vi "Camera Loop.vi"(6 "Used functions":bool=TRUE, 8 "error in":errorcluster, 9 "IBM OptoElectroMechanics Configuration":T1={"Parameter Analizer"={"Parameter Analyzer VISA Session"="COM1", "Sweeping Time Parameters"={"Integration Time"=0, "Short Integration Time (s)"=1.0, "Long Integration Time (s)"=0.0, "Wait Time Parameter"=1.0}, "Acquisition Mode"=enum."Sweeping Mode", "Status Polling Time (ms)"=0, "Comment"="Test VI", "SMU 1 - Sweeping"={"Start / Offset"=0.0, "Stop / Ratio"=1.0, "Step \n(linear only)"=0.01, "Compliance"=0.1, "Power \nCompliance"=0.0, "Mode"=0, "Function"=0, "Sweep Mode"=FALSE}, "SMU 2 - Sweeping"={"Start / Offset"=0.0, "Stop / Ratio"=1.0, "Step \n(linear only)"=0.01, "Compliance"=0.1, "Power \nCompliance"=0.0, "Mode"=0, "Function"=0, "Sweep Mode"=FALSE}, "SMU 3 - Sweeping"={"Start / Offset"=0.0, "Stop / Ratio"=1.0, "Step \n(linear only)"=0.01, "Compliance"=0.1, "Power \nCompliance"=0.0, "Mode"=0, "Function"=0, "Sweep Mode"=FALSE}, "SMU 4 - Sweeping"={"Start / Offset"=0.0, "Stop / Ratio"=1.0, "Step \n(linear only)"=0.01, "Compliance"=0.1, "Power \nCompliance"=0.0, "Mode"=0, "Function"=0, "Sweep Mode"=FALSE}, "Sweep Spacing"=0, "Range"=0, "SMU1 - Sampling"={"Source"=10.0, "Compliance"=1e-05, "Mode"=0, "Function"=FALSE}, "SMU2 - Sampling"={"Source"=1.0, "Compliance"=1.0, "Mode"=0, "Function"=FALSE}, "SMU3 - Sampling"={"Source"=10.0, "Compliance"=1e-05, "Mode"=0, "Function"=FALSE}, "SMU4 - Sampling"={"Source"=0.1, "Compliance"=60.0, "Mode"=10, "Function"=FALSE}, "Sampling Time Parameters"={"Initial Interval (s)"=0.1, "Number of Samples"=60, "Total Sampling Time (s)"=10.0, "Hold Time (s)"=0.0, "Sampling Mode"=0, "Sampling Time"=0}, "Stop Condition"={"Enable Delay (s)"=0.0, "Name"="", "Threshold"=0.0, "num. of events"=1, "Event"=0, "Stop Condition Enable"=FALSE}}, "Switching Matrix"={"Switching Matrix VISA Session"="GPIB0::18::INSTR", "Connections"=[{"Connections"=[FALSE, FALSE, FALSE, FALSE, FALSE, FALSE, FALSE, FALSE, FALSE, FALSE, FALSE, FALSE], "Connection Type"=enum."Disconnected"}, {"Connections"=[FALSE, FALSE, FALSE, FALSE, FALSE, FALSE, FALSE, FALSE, FALSE, FALSE, FALSE, FALSE], "Connection Type"=enum."Disconnected"}, {"Connections"=[FALSE, FALSE, FALSE, FALSE, FALSE, FALSE, FALSE, FALSE, FALSE, FALSE, FALSE, FALSE], "Connection Type"=enum."Disconnected"}, {"Connections"=[FALSE, FALSE, FALSE, FALSE, FALSE, FALSE, FALSE, FALSE, FALSE, FALSE, FALSE, FALSE], "Connection Type"=enum."Disconnected"}, {"Connections"=[FALSE, FALSE, FALSE, FALSE, FALSE, FALSE, FALSE, FALSE, FALSE, FALSE, FALSE, FALSE], "Connection Type"=enum."Disconnected"}, {"Connections"=[FALSE, FALSE, FALSE, FALSE, FALSE, FALSE, FALSE, FALSE, FALSE, FALSE, FALSE, FALSE], "Connection Type"=enum."Disconnected"}, {"Connections"=[FALSE, FALSE, FALSE, FALSE, FALSE, FALSE, FALSE, FALSE, FALSE, FALSE, FALSE, FALSE], "Connection Type"=enum."Disconnected"}, {"Connections"=[FALSE, FALSE, FALSE, FALSE, FALSE, FALSE, FALSE, FALSE, FALSE, FALSE, FALSE, FALSE], "Connection Type"=enum."Disconnected"}]}, "Stress Control"={"Stress Control VISA Session"="StrainMotor", "Axis"=0, "Motion"=0, "Destination (°)"=0.0, "Speed (°/s)"=4.0, "Position (°)"=25.0}, "Optical Spectrometer"={"Laser Settings"={"Laser Wavelength"=enum."365 nm", "Neutral Density Filter"=enum."100%"}, "Spectrometer Settings"={"Confocal Hole Size (µm)"=0.0, "Grating"=2, "Detector"=enum."InGaAs Array"}, "Acquisition Settings"={"Acquisition Mode"=enum."Multi-Window", "Spectal Position (nm)"=632.0, "From (nm)"=735.0, "To (nm)"=0.0, "Integration Time (s)"=0.0, "Number of Accumulations"=3, "AutoScanning"=FALSE, "Spike Removal"=FALSE}, "Path"=path "C:/07 - Prizes and Awards/Marie Curie Prize/Reply Editors Final NCOMMS(10).docx"}, "Switches & Mirrors"={"Relay VISA Session"="COM1", "Switches"={"Laser"=FALSE, "Video"=FALSE}, "Delays (ms)"={"Laser"=500, "Video"=1500}}, "Camera"={"Settings"={"Pixel clock"=20, "Frame rate"=30.0, "Exposure time"=33.21525, "Master Gain"=0, "Red Gain"=0, "Green Gain"=0, "Blue Gain"=0, "Auto Gain"=FALSE, "White-balance"=FALSE, "Color Correction"=FALSE}}, "XYZ Stage"={"Connection Settings"={"Tango VISA"="", "Baudrate"=57600, "Show Protocol?"=FALSE}, "Manual Control"={"North"=FALSE, "South"=FALSE, "West"=FALSE, "East"=FALSE, "Up"=FALSE, "Down"=FALSE, "Stop"=FALSE, "XY Step"=0.0, "Z step"=0.0}, "Coordinate Control"={"Motion Mode"=enum."Absolute", "Destination [mm]"=[]}}, "AutoFocus"={"Matching Criteria"={"Minimum Score"=700.0, "Color Score Weight"=700.0, "Minimum Contrast"=50, "Match Mode"=0, "Match Feature Mode"=0, "Subpixel Accuracy"=TRUE, "Color Sensitivity"=1, "Search Strategy"=1}, "Z Scan Parameters"={"Z Range"=1380.0, "Resolution"=5000.0, "Initial Direction"=enum."Up", "Focus Threshold"=0.1, "Ascent Constant"=0.1}, "Displacement"=0.0, "Transformation Matrix"=[]}, "Sava Data"={"Workspace Info"={"Device Name"="ProberHead_Tst_C29K3_7(2)", "Device Info"="ProberHead_Tst_C29", "Path"=path "C:/Users/gio/Desktop/ProbeHeadTest"}, "Instrument Configuration"={"Instrument"=enum."Unknown Instrument", "Configuration"="Test Configuration"}, "Stress Motor Position"=0.0, "Electrical Measurement"={"Sequence"=[], "V1"=[], "V2"=[], "V3"=[], "V4"=[], "I1"=[], "I2"=[], "I3"=[], "I4"=[]}, "Optical Spectrum"={"Intensity"=[], "Wavelength"=[], "Energy"=[], "Raman Shift"=[], "Detector Temperature"=0.0}}, "PlotData"={"Sliders"={"Strain Sequence"=0, "Instrument Sequence"=0}, "Measurement"={"Which Instrument?"=enum."No Plot", "Electrical Measurement"={"Sequence"=[], "V1"=[], "V2"=[], "V3"=[], "V4"=[], "I1"=[], "I2"=[], "I3"=[], "I4"=[]}, "Measurement Mode"=enum."Sweeping Mode", "Optical Spectrum"={"Intensity"=[], "Wavelength"=[], "Energy"=[], "Raman Shift"=[], "Detector Temperature"=0.0}}, "Instrument Steps"=[], "Strain Points"=[]}, "Instrument Sequence"={"Caller VI"=enum."User"}, "Strain Measurement"={"Stress Sequence "={"Max Motor Position"=1380.0, "# Intermediate Points"=5000, "Initial Direction"=enum."Tension"}, "Track?"=FALSE}} {"AutoFocus"."Displacement" scale=1.0..1000.0; "AutoFocus"."Z Scan Parameters"."Focus Threshold" min=0.0 max=1000.0 step=1.0 format="%#_2f"; "AutoFocus"."Z Scan Parameters"."Ascent Constant" min=0.0 max=1000.0 step=1.0 format="%#_2f"; "AutoFocus"."Z Scan Parameters"."Resolution" min=0.0 max=1.0 step=0.01 format="%_2g"; "AutoFocus"."Z Scan Parameters"."Z Range" format="%_3g"; "AutoFocus"."Matching Criteria"."Match Mode" items=["Shift Invariant", "Rotation Invariant"]; "AutoFocus"."Matching Criteria"."Match Feature Mode" items=["Color and Shape", "Color", "Shape"]; "AutoFocus"."Matching Criteria"."Color Sensitivity" items=["Low Sensitivity", "Medium Sensitivity", "High Sensitivity"]; "AutoFocus"."Matching Criteria"."Search Strategy" items=["Conservative", "Balance", "Aggressive", "Very Aggressive"]; "XYZ Stage"."Manual Control"."Z step" scale=0.1..10.0; "XYZ Stage"."Manual Control"."XY Step" scale=0.1..1000.0; "Camera"."Settings"."Blue Gain" min=0 max=100 scale=0.0..100.0; "Camera"."Settings"."Green Gain" min=0 max=100 scale=0.0..100.0; "Camera"."Settings"."Red Gain" min=0 max=100 scale=0.0..100.0; "Camera"."Settings"."Master Gain" min=0 max=100 scale=0.0..100.0; "Camera"."Settings"."Exposure time" min=0.101625 max=159.246375 step=0.101625 scale=0.101625..159.246375 scale format="%#.3g"; "Camera"."Settings"."Frame rate" min=2.7455631699174137 max=6.2675785993528725 step=0.000101625 scale=2.7455631699174137..6.2675785993528725 scale format="%^#_3g"; "Camera"."Settings"."Pixel clock" min=5 max=43 scale=5.0..43.0; "PlotData"."Sliders"."Instrument Sequence" scale=0.0..10.0; "PlotData"."Sliders"."Strain Sequence" scale=0.0..10.0; "Strain Measurement"."Stress Sequence"."# Intermediate Points" max=1390; "Parameter Analizer"."Stop Condition"."Event" items=["Value > Threshold", "Value < Threshold", "| Value | > | Threshold |", "| Value | < | Threshold |"]; "Parameter Analizer"."Stop Condition"."Threshold" format="%^.2e"; "Parameter Analizer"."Stop Condition"."Enable Delay (s)" format="%.1f"; "Parameter Analizer"."Sampling Time Parameters"."Sampling Time" items=["Auto (linear only)", "No Limit", "Set Limit"]; "Parameter Analizer"."Sampling Time Parameters"."Sampling Mode" items=["Linear", "Log10", "Log25", "Log50", "Thinned Out"]; "Parameter Analizer"."Sampling Time Parameters"."Hold Time (s)" format="%.4f"; "Parameter Analizer"."Sampling Time Parameters"."Total Sampling Time (s)" format="%.1f"; "Parameter Analizer"."Sampling Time Parameters"."Initial Interval (s)" format="%^.3e"; "Parameter Analizer"."SMU 4 - Sweeping"."Function" items=["Disabled", "Var 1", "Var 2", "Var 1'", "Constant"]; "Parameter Analizer"."SMU 4 - Sweeping"."Mode" items=["V", "I", "V pulse", "I  pulse", "Common"]; "Parameter Analizer"."SMU 4 - Sweeping"."Power \nCompliance" format="%^.2e"; "Parameter Analizer"."SMU 4 - Sweeping"."Compliance" format="%^.2e"; "Parameter Analizer"."SMU 4 - Sweeping"."Step \n(linear only)" format="%^.4e"; "Parameter Analizer"."SMU 4 - Sweeping"."Stop / Ratio" format="%^.4e"; "Parameter Analizer"."SMU 4 - Sweeping"."Start / Offset" format="%^.4e"; "Parameter Analizer"."SMU 3 - Sweeping"."Function" items=["Disabled", "Var 1", "Var 2", "Var 1'", "Constant"]; "Parameter Analizer"."SMU 3 - Sweeping"."Mode" items=["V", "I", "V pulse", "I  pulse", "Common"]; "Parameter Analizer"."SMU 3 - Sweeping"."Power \nCompliance" format="%^.2e"; "Parameter Analizer"."SMU 3 - Sweeping"."Compliance" format="%^.2e"; "Parameter Analizer"."SMU 3 - Sweeping"."Step \n(linear only)" format="%^.4e"; "Parameter Analizer"."SMU 3 - Sweeping"."Stop / Ratio" format="%^.4e"; "Parameter Analizer"."SMU 3 - Sweeping"."Start / Offset" format="%^.4e"; "Parameter Analizer"."SMU 2 - Sweeping"."Function" items=["Disabled", "Var 1", "Var 2", "Var 1'", "Constant"]; "Parameter Analizer"."SMU 2 - Sweeping"."Mode" items=["V", "I", "V pulse", "I  pulse", "Common"]; "Parameter Analizer"."SMU 2 - Sweeping"."Power \nCompliance" format="%^.2e"; "Parameter Analizer"."SMU 2 - Sweeping"."Compliance" format="%^.2e"; "Parameter Analizer"."SMU 2 - Sweeping"."Step \n(linear only)" format="%^.4e"; "Parameter Analizer"."SMU 2 - Sweeping"."Stop / Ratio" format="%^.4e"; "Parameter Analizer"."SMU 2 - Sweeping"."Start / Offset" format="%^.4e"; "Parameter Analizer"."SMU 1 - Sweeping"."Function" items=["Disabled", "Var 1", "Var 2", "Var 1'", "Constant"]; "Parameter Analizer"."SMU 1 - Sweeping"."Mode" items=["V", "I", "V pulse", "I  pulse", "Common"]; "Parameter Analizer"."SMU 1 - Sweeping"."Power \nCompliance" format="%^.2e"; "Parameter Analizer"."SMU 1 - Sweeping"."Compliance" format="%^.2e"; "Parameter Analizer"."SMU 1 - Sweeping"."Step \n(linear only)" format="%^.4e"; "Parameter Analizer"."SMU 1 - Sweeping"."Stop / Ratio" format="%^.4e"; "Parameter Analizer"."SMU 1 - Sweeping"."Start / Offset" format="%^.4e"; "Parameter Analizer"."Sweeping Time Parameters"."Long Integration Time (s)" scale=0.02..2.0; "Parameter Analizer"."Sweeping Time Parameters"."Short Integration Time (s)" scale=8e-05..0.00192; "Parameter Analizer"."Sweeping Time Parameters"."Integration Time" items=["Short", "Long"]; "Parameter Analizer"."Sweeping Time Parameters"."Wait Time Parameter" format="%.1f"; "Parameter Analizer"."SMU4 - Sampling"."Mode" items=["V", "I", "Common"]; "Parameter Analizer"."SMU4 - Sampling"."Compliance" format="%^.2e"; "Parameter Analizer"."SMU4 - Sampling"."Source" format="%^.3e"; "Parameter Analizer"."SMU3 - Sampling"."Mode" items=["V", "I", "Common"]; "Parameter Analizer"."SMU3 - Sampling"."Compliance" format="%^.2e"; "Parameter Analizer"."SMU3 - Sampling"."Source" format="%^.3e"; "Parameter Analizer"."SMU2 - Sampling"."Mode" items=["V", "I", "Common"]; "Parameter Analizer"."SMU2 - Sampling"."Compliance" format="%^.2e"; "Parameter Analizer"."SMU2 - Sampling"."Source" format="%^.3e"; "Parameter Analizer"."SMU1 - Sampling"."Mode" items=["V", "I", "Common"]; "Parameter Analizer"."SMU1 - Sampling"."Compliance" format="%^.2e"; "Parameter Analizer"."SMU1 - Sampling"."Source" format="%^.3e"; "Parameter Analizer"."Range" items=["auto", "fixed", "limited"]; "Parameter Analizer"."Sweep Spacing" items=["linear", "log 10", "log 25", "log 50"]; "Stress Control"."Axis" min=1 max=3; "Stress Control"."Position (°)" format="%.6g"; "Stress Control"."Speed (°/s)" min=0.0 max=4.0 format="%.6f"; "Stress Control"."Destination (°)" min=-2000000000.0 max=2000000000.0 format="%.6f"; "Stress Control"."Motion" items=["Absolute", "Relative"]; "Optical Spectrometer"."Spectrometer Settings"."Grating" items=["1800 l/mm", "150 l/mm"]}, 10 "Message Queues out":T57, 11 "Notifiers":T44) -> (0 "error out":errorcluster)   [LabVIEW 2014]
uses:
  support/Message Queue/All Message Queues.ctl
  support/Message Queue/Message Cluster.ctl
  support/Notifiers/Notifiers.ctl
  support/Message Handler Loop Notifiers.ctl
  Hardware Control/Parameter Analyzer/Parameter Analyzer Notifiers.ctl
  Hardware Control/Switching Matrix/Switching Matrix Notifiers.ctl
  Hardware Control/Stress Control/StressControl Notifiers.ctl
  Hardware Control/Spectrometer/Spectrometer Notifiers.ctl
  Hardware Control/Switches and Mirrors/SwitchesMirrors Notifiers.ctl
  Hardware Control/Camera/Camera Notifiers.ctl
  Hardware Control/XYZ Stage/XYZ Notifications.ctl
  Hardware Control/Autofocus/Autofocus Notifiers.ctl
  Measurements/Optoelectronic Measurement/Optoelectronic Notifiers.ctl
  Measurements/Save Data/SaveData Notifiers.ctl
  Measurements/Instrument Sequence/Instrument Sequence Notifiers.ctl
  support/Configuration/Configuration.ctl
  Hardware Control/Parameter Analyzer/Parameter Analyzer Config.ctl
  Hardware Control/Parameter Analyzer/Parameter Analyzer Integration Parameters.ctl
  Hardware Control/Parameter Analyzer/Parameter Analyzer SMU Sweeping.ctl
  Hardware Control/Parameter Analyzer/Parameter Analyzer Sweep Spacing.ctl
  Hardware Control/Parameter Analyzer/Parameter Analyzer SMU Range.ctl
  Hardware Control/Parameter Analyzer/Parameter Analyzer SMU Sampling.ctl
  Hardware Control/Parameter Analyzer/Parameter Analyzer Sampling Parameters.ctl
  Hardware Control/Parameter Analyzer/Parameter Analyzer Stop Sampling Conditions.ctl
  Hardware Control/Switching Matrix/Switching Matrix Config.ctl
  Hardware Control/Stress Control/StressControl Config.ctl
  Hardware Control/Spectrometer/Spectrometer Config.ctl
  Hardware Control/Spectrometer/Laser Settings.ctl
  Hardware Control/Spectrometer/Laser.ctl
  Hardware Control/Spectrometer/Filter.ctl
  Hardware Control/Spectrometer/Grating Detector Settings.ctl
  Hardware Control/Spectrometer/Grating.ctl
  Hardware Control/Spectrometer/Detector.ctl
  Hardware Control/Spectrometer/Acquisition Settings.ctl
  Hardware Control/Switches and Mirrors/SwitchesMirrors Config.ctl
  Hardware Control/Switches and Mirrors/SwitchesMirrors Status.ctl
  Hardware Control/Camera/Camera Config.ctl
  Hardware Control/Camera/Camera Settings.ctl
  Hardware Control/XYZ Stage/XYZ Config.ctl
  Hardware Control/XYZ Stage/XYZ Connection Settings.ctl
  Hardware Control/XYZ Stage/XYZ Stage Control.ctl
  Hardware Control/XYZ Stage/XYZ Coordinate Control.ctl
  Hardware Control/Autofocus/AutoFocus Config.ctl
  Hardware Control/Autofocus/ZScan.ctl
  <vilib>/Analysis/Matrix/Datatypes/RealMatrix.ctl
  Measurements/Save Data/SaveData Config.ctl
  Measurements/Save Data/SaveData Workspace Info.ctl
  Measurements/Save Data/SaveData Instrument Configuration.ctl
  Measurements/Instrument Sequence/Instrument List.ctl
  Hardware Control/Spectrometer/Spectral Data.ctl
  Measurements/Plot Data/PlotData Config.ctl
  Measurements/Plot Data/Measurement.ctl
  Measurements/Plot Data/WhichInstrument.ctl
  Hardware Control/Parameter Analyzer/Electrical Data.ctl
  Measurements/Instrument Sequence/Instrument Steps.ctl
  Measurements/Instrument Sequence/Action.ctl
  Measurements/Instrument Sequence/Instrument Sequence Config.ctl
  Measurements/Strain Measurement/Strain Measurement Config.ctl
  Hardware Control/Camera/Camera Functions.ctl
  support/Message Queue/Message Queue.lvlib
  <vilib>/Analysis/Matrix/NI_Matrix.lvlib
panel:
  # "LICENSED MATERIALS – PROPERTY OF IBM\nCopyright IBM Corp. 2016,\nALL RIGHTS RESERVED"
  # "XY"
  # "Z"
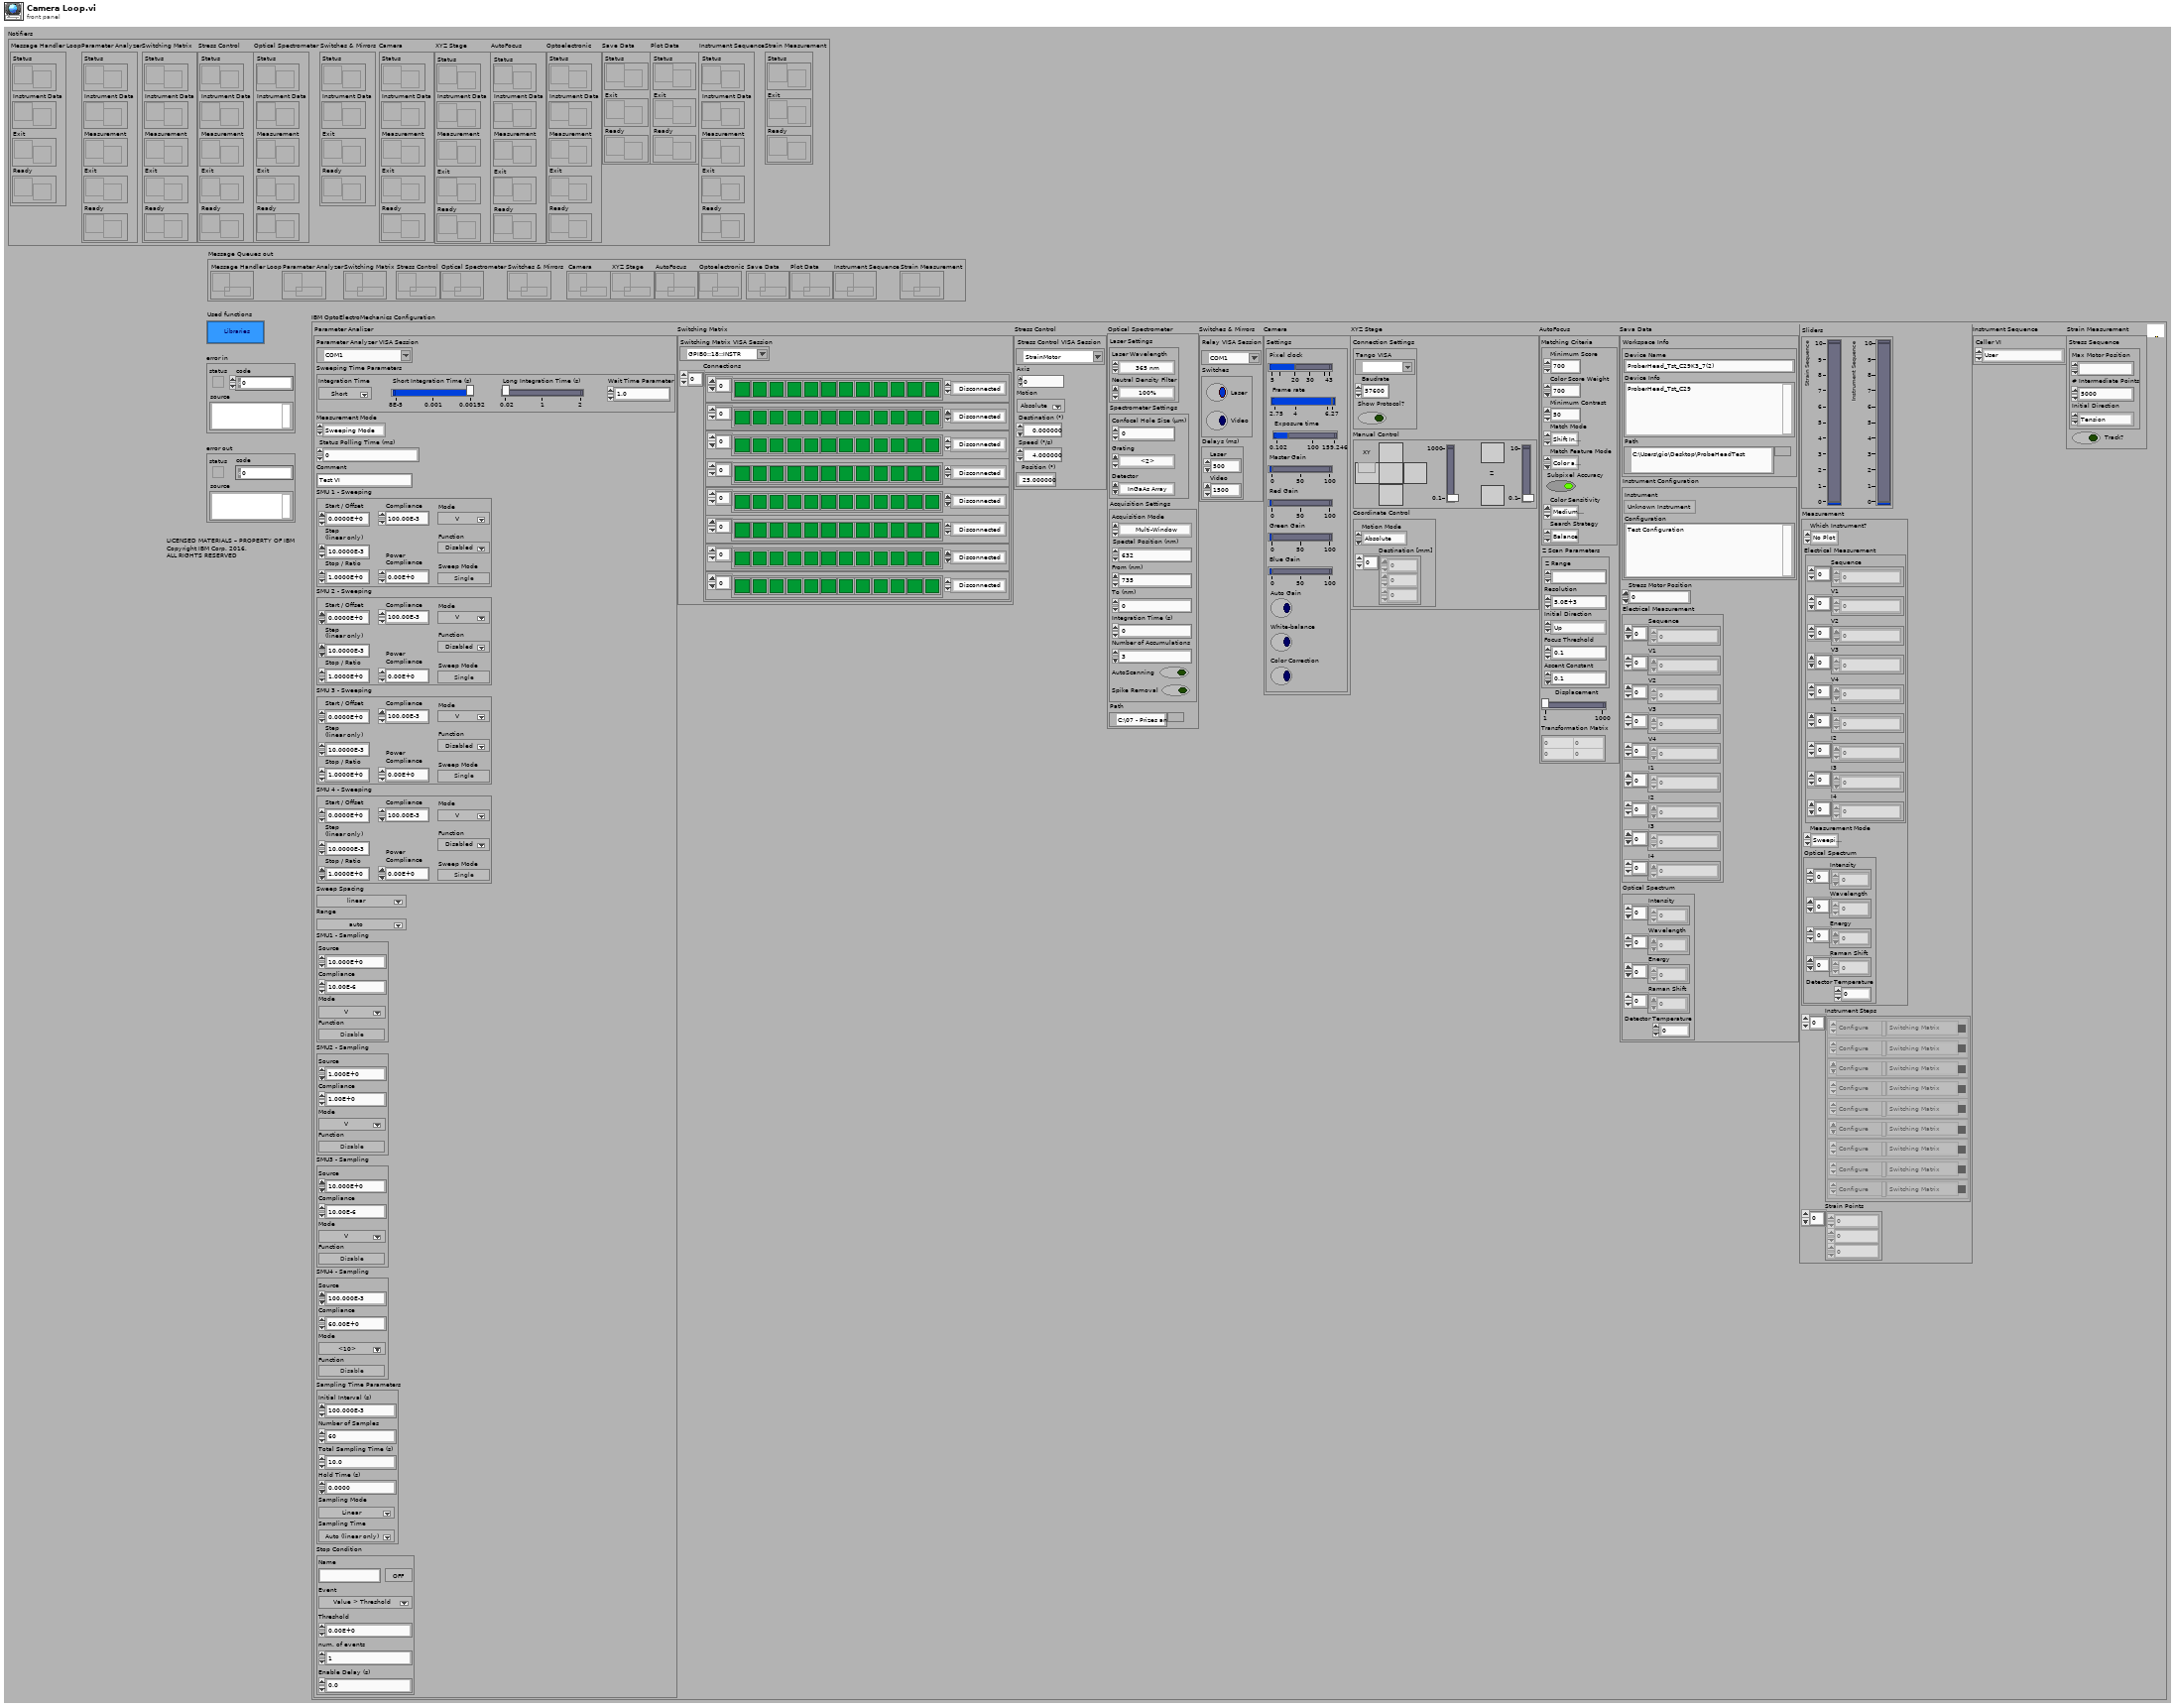
[diagram p1: front panel]
types:
  T1 = typedef "Configuration.ctl" = cluster{"Parameter Analizer":T2, "Switching Matrix":T10, "Stress Control":T11, "Optical Spectrometer":T12, "Switches & Mirrors":T20, "Camera":T22, "XYZ Stage":T24, "AutoFocus":T28, "Sava Data":T31, "PlotData":T36, "Instrument Sequence":T42, "Strain Measurement":T43}
  T2 = typedef "Parameter Analyzer Config.ctl" = cluster{"Parameter Analyzer VISA Session":refnum<visa-resource-name>, "Sweeping Time Parameters":T3, "Acquisition Mode":enum32{"Sweeping Mode", "Sampling Mode"}, "Status Polling Time (ms)":u32, "Comment":string, "SMU 1 - Sweeping":T4, "SMU 2 - Sweeping":T4, "SMU 3 - Sweeping":T4, "SMU 4 - Sweeping":T4, "Sweep Spacing":T5, "Range":T6, "SMU1 - Sampling":T7, "SMU2 - Sampling":T7, "SMU3 - Sampling":T7, "SMU4 - Sampling":T7, "Sampling Time Parameters":T8, "Stop Condition":T9}
  T3 = typedef "Parameter Analyzer Integration Parameters.ctl" = cluster{"Integration Time":u32, "Short Integration Time (s)":dbl, "Long Integration Time (s)":dbl, "Wait Time Parameter":dbl}
  T4 = typedef "Parameter Analyzer SMU Sweeping.ctl" = cluster{"Start / Offset":dbl, "Stop / Ratio":dbl, "Step \n(linear only)":dbl, "Compliance":dbl, "Power \nCompliance":dbl, "Mode":u32, "Function":i32, "Sweep Mode":bool}
  T5 = typedef "Parameter Analyzer Sweep Spacing.ctl" = u16
  T6 = typedef "Parameter Analyzer SMU Range.ctl" = u16
  T7 = typedef "Parameter Analyzer SMU Sampling.ctl" = cluster{"Source":dbl, "Compliance":dbl, "Mode":u32, "Function":bool}
  T8 = typedef "Parameter Analyzer Sampling Parameters.ctl" = cluster{"Initial Interval (s)":dbl, "Number of Samples":i32, "Total Sampling Time (s)":dbl, "Hold Time (s)":dbl, "Sampling Mode":i32, "Sampling Time":i32}
  T9 = typedef "Parameter Analyzer Stop Sampling Conditions.ctl" = cluster{"Enable Delay (s)":dbl, "Name":string, "Threshold":dbl, "num. of events":i32, "Event":i32, "Stop Condition Enable":bool}
  T10 = typedef "Switching Matrix Config.ctl" = cluster{"Switching Matrix VISA Session":refnum<visa-resource-name>, "Connections":cluster{"Connections":bool[], "Connection Type":enum16{"Disconnected", "Make - Break", "Break - Make"}}[]}
  T11 = typedef "StressControl Config.ctl" = cluster{"Stress Control VISA Session":refnum<visa-resource-name>, "Axis":i32, "Motion":u16, "Destination (°)":dbl, "Speed (°/s)":dbl, "Position (°)":dbl}
  T12 = typedef "Spectrometer Config.ctl" = cluster{"Laser Settings":T13, "Spectrometer Settings":T16, "Acquisition Settings":T19, "Path":path}
  T13 = typedef "Laser Settings.ctl" = cluster{"Laser Wavelength":T14, "Neutral Density Filter":T15}
  T14 = typedef "Laser.ctl" = enum16{"633 nm", "784 nm", "532 nm", "365 nm"}
  T15 = typedef "Filter.ctl" = enum16{"100%", "50%", "25%", "10%", "1%", "0.1%", "0.01%"}
  T16 = typedef "Grating Detector Settings.ctl" = cluster{"Confocal Hole Size (µm)":dbl, "Grating":T17, "Detector":T18}
  T17 = typedef "Grating.ctl" = u16
  T18 = typedef "Detector.ctl" = enum16{"InGaAs Array", "Silicon CCD"}
  T19 = typedef "Acquisition Settings.ctl" = cluster{"Acquisition Mode":enum16{"Single Window", "Multi-Window"}, "Spectal Position (nm)":dbl, "From (nm)":dbl, "To (nm)":dbl, "Integration Time (s)":dbl, "Number of Accumulations":i32, "AutoScanning":bool, "Spike Removal":bool}
  T20 = typedef "SwitchesMirrors Config.ctl" = cluster{"Relay VISA Session":refnum<visa-resource-name>, "Switches":T21, "Delays (ms)":cluster{"Laser":u32, "Video":u32}}
  T21 = typedef "SwitchesMirrors Status.ctl" = cluster{"Laser":bool, "Video":bool}
  T22 = typedef "Camera Config.ctl" = cluster{"Settings":T23}
  T23 = typedef "Camera Settings.ctl" = cluster{"Pixel clock":i32, "Frame rate":dbl, "Exposure time":dbl, "Master Gain":i32, "Red Gain":i32, "Green Gain":i32, "Blue Gain":i32, "Auto Gain":bool, "White-balance":bool, "Color Correction":bool}
  T24 = typedef "XYZ Config.ctl" = cluster{"Connection Settings":T25, "Manual Control":T26, "Coordinate Control":T27}
  T25 = typedef "XYZ Connection Settings.ctl" = cluster{"Tango VISA":refnum<visa-resource-name>, "Baudrate":i32, "Show Protocol?":bool}
  T26 = typedef "XYZ Stage Control.ctl" = cluster{"North":bool, "South":bool, "West":bool, "East":bool, "Up":bool, "Down":bool, "Stop":bool, "XY Step":dbl, "Z step":dbl}
  T27 = typedef "XYZ Coordinate Control.ctl" = cluster{"Motion Mode":enum16{"Absolute", "Relative"}, "Destination [mm]":dbl[]}
  T28 = typedef "AutoFocus Config.ctl" = cluster{"Matching Criteria":cluster{"Minimum Score":sgl, "Color Score Weight":sgl, "Minimum Contrast":i32, "Match Mode":u32, "Match Feature Mode":u32, "Subpixel Accuracy":bool, "Color Sensitivity":u32, "Search Strategy":u32}, "Z Scan Parameters":T29, "Displacement":dbl, "Transformation Matrix":T30}
  T29 = typedef "ZScan.ctl" = cluster{"Z Range":ext, "Resolution":dbl, "Initial Direction":enum16{"Up", "Down"}, "Focus Threshold":dbl, "Ascent Constant":dbl}
  T30 = typedef "NI_Matrix.lvlib/RealMatrix.ctl" = dbl[][]
  T31 = typedef "SaveData Config.ctl" = cluster{"Workspace Info":T32, "Instrument Configuration":T33, "Stress Motor Position":dbl, "Electrical Measurement":cluster{"Sequence":dbl[], "V1":dbl[], "V2":dbl[], "V3":dbl[], "V4":dbl[], "I1":dbl[], "I2":dbl[], "I3":dbl[], "I4":dbl[]}, "Optical Spectrum":T35}
  T32 = typedef "SaveData Workspace Info.ctl" = cluster{"Device Name":string, "Device Info":string, "Path":path}
  T33 = typedef "SaveData Instrument Configuration.ctl" = cluster{"Instrument":T34, "Configuration":string}
  T34 = typedef "Instrument List.ctl" = enum32{"Unknown Instrument", "Switching Matrix", "Parameter Analyzer", "Optical Spectrometer", "Optoelectronic", "Autofocus"}
  T35 = typedef "Spectral Data.ctl" = cluster{"Intensity":dbl[], "Wavelength":dbl[], "Energy":dbl[], "Raman Shift":dbl[], "Detector Temperature":dbl}
  T36 = typedef "PlotData Config.ctl" = cluster{"Sliders":cluster{"Strain Sequence":i32, "Instrument Sequence":i32}, "Measurement":T37, "Instrument Steps":T40, "Strain Points":dbl[]}
  T37 = typedef "Measurement.ctl" = cluster{"Which Instrument?":T38, "Electrical Measurement":T39, "Measurement Mode":enum16{"Sweeping Mode", "Sampling Mode"}, "Optical Spectrum":T35}
  T38 = typedef "WhichInstrument.ctl" = enum16{"No Plot", "Spectrometer", "Parameter Analyzer", "Optoelectronic"}
  T39 = typedef "Electrical Data.ctl" = cluster{"Sequence":dbl[], "V1":dbl[], "V2":dbl[], "V3":dbl[], "V4":dbl[], "I1":dbl[], "I2":dbl[], "I3":dbl[], "I4":dbl[]}
  T40 = typedef "Instrument Steps.ctl" = cluster{"Action":T41, "Configuration":variant, "Instrument":T34, "Status":enum8{"False", "True", "Mixed"}}[]
  T41 = typedef "Action.ctl" = enum32{"Configure", "Measure"}
  T42 = typedef "Instrument Sequence Config.ctl" = cluster{"Caller VI":enum16{"User", "Stress Measurement VI"}}
  T43 = typedef "Strain Measurement Config.ctl" = cluster{"Stress Sequence ":cluster{"Max Motor Position":ext, "# Intermediate Points":u32, "Initial Direction":enum16{"Tension", "Compression"}}, "Track?":bool}
  T44 = typedef "Notifiers.ctl" = cluster{"Message Handler Loop":T45, "Parameter Analyzer":T46, "Switching Matrix":T47, "Stress Control":T48, "Optical Spectrometer":T49, "Switches & Mirrors":T50, "Camera":T51, "XYZ Stage":T52, "AutoFocus":T53, "Optoelectronic":T54, "Save Data":T55, "Plot Data":T55, "Instrument Sequence":T56, "Strain Measurement":cluster{"Status":refnum<notifier>, "Exit":refnum<notifier>, "Ready":refnum<notifier>}}
  T45 = typedef "Message Handler Loop Notifiers.ctl" = cluster{"Status":refnum<notifier>, "Instrument Data":refnum<notifier>, "Exit":refnum<notifier>, "Ready":refnum<notifier>}
  T46 = typedef "Parameter Analyzer Notifiers.ctl" = cluster{"Status":refnum<notifier>, "Instrument Data":refnum<notifier>, "Measurement":refnum<notifier>, "Exit":refnum<notifier>, "Ready":refnum<notifier>}
  T47 = typedef "Switching Matrix Notifiers.ctl" = cluster{"Status":refnum<notifier>, "Instrument Data":refnum<notifier>, "Measurement":refnum<notifier>, "Exit":refnum<notifier>, "Ready":refnum<notifier>}
  T48 = typedef "StressControl Notifiers.ctl" = cluster{"Status":refnum<notifier>, "Instrument Data":refnum<notifier>, "Measurement":refnum<notifier>, "Exit":refnum<notifier>, "Ready":refnum<notifier>}
  T49 = typedef "Spectrometer Notifiers.ctl" = cluster{"Status":refnum<notifier>, "Instrument Data":refnum<notifier>, "Measurement":refnum<notifier>, "Exit":refnum<notifier>, "Ready":refnum<notifier>}
  T50 = typedef "SwitchesMirrors Notifiers.ctl" = cluster{"Status":refnum<notifier>, "Instrument Data":refnum<notifier>, "Exit":refnum<notifier>, "Ready":refnum<notifier>}
  T51 = typedef "Camera Notifiers.ctl" = cluster{"Status":refnum<notifier>, "Instrument Data":refnum<notifier>, "Measurement":refnum<notifier>, "Exit":refnum<notifier>, "Ready":refnum<notifier>}
  T52 = typedef "XYZ Notifications.ctl" = cluster{"Status":refnum<notifier>, "Instrument Data":refnum<notifier>, "Measurement":refnum<notifier>, "Exit":refnum<notifier>, "Ready":refnum<notifier>}
  T53 = typedef "Autofocus Notifiers.ctl" = cluster{"Status":refnum<notifier>, "Instrument Data":refnum<notifier>, "Measurement":refnum<notifier>, "Exit":refnum<notifier>, "Ready":refnum<notifier>}
  T54 = typedef "Optoelectronic Notifiers.ctl" = cluster{"Status":refnum<notifier>, "Instrument Data":refnum<notifier>, "Measurement":refnum<notifier>, "Exit":refnum<notifier>, "Ready":refnum<notifier>}
  T55 = typedef "SaveData Notifiers.ctl" = cluster{"Status":refnum<notifier>, "Exit":refnum<notifier>, "Ready":refnum<notifier>}
  T56 = typedef "Instrument Sequence Notifiers.ctl" = cluster{"Status":refnum<notifier>, "Instrument Data":refnum<notifier>, "Measurement":refnum<notifier>, "Exit":refnum<notifier>, "Ready":refnum<notifier>}
  T57 = typedef "Message Queue.lvlib/All Message Queues.ctl" = cluster{"Message Handler Loop":refnum<queue>, "Parameter Analyzer":refnum<queue>, "Switching Matrix":refnum<queue>, "Stress Control":refnum<queue>, "Optical Spectrometer":refnum<queue>, "Switches & Mirrors":refnum<queue>, "Camera":refnum<queue>, "XYZ Stage":refnum<queue>, "AutoFocus":refnum<queue>, "Optoelectronic":refnum<queue>, "Save Data":refnum<queue>, "Plot Data":refnum<queue>, "Instrument Sequence":refnum<queue>, "Strain Measurement":refnum<queue>}
  T58 = typedef "Camera Data.ctl" = cluster{"Configuration":T22, "Refnums":T59, "Initialization":T60}
  T59 = typedef "Camera Refnums.ctl" = cluster{"Pixel Clock":refnum<vi>, "Frame Rate":refnum<vi>, "Exposure Time":refnum<vi>, "Master Gain":refnum<vi>, "Red Gain":refnum<vi>, "Green Gain":refnum<vi>, "Blue Gain":refnum<vi>, "Auto Gain":refnum<vi>, "Auto White-balance":refnum<vi>, "Color Correction":refnum<vi>, "Image":refnum<vi>, "Video Button":refnum<vi>, "Instrument Status":refnum<vi>}
  T60 = typedef "Camera Initialization.ctl" = cluster{"Connect":bool, "Update Refnums":bool, "Acquiring?":bool}
  T61 = typedef "Camera Functions.ctl" = enum16{"Connect", "Start Live", "Acquire", "Update Settings", "Update Settings2", "Stop Live", "Disconnect", "Update Refnums"}
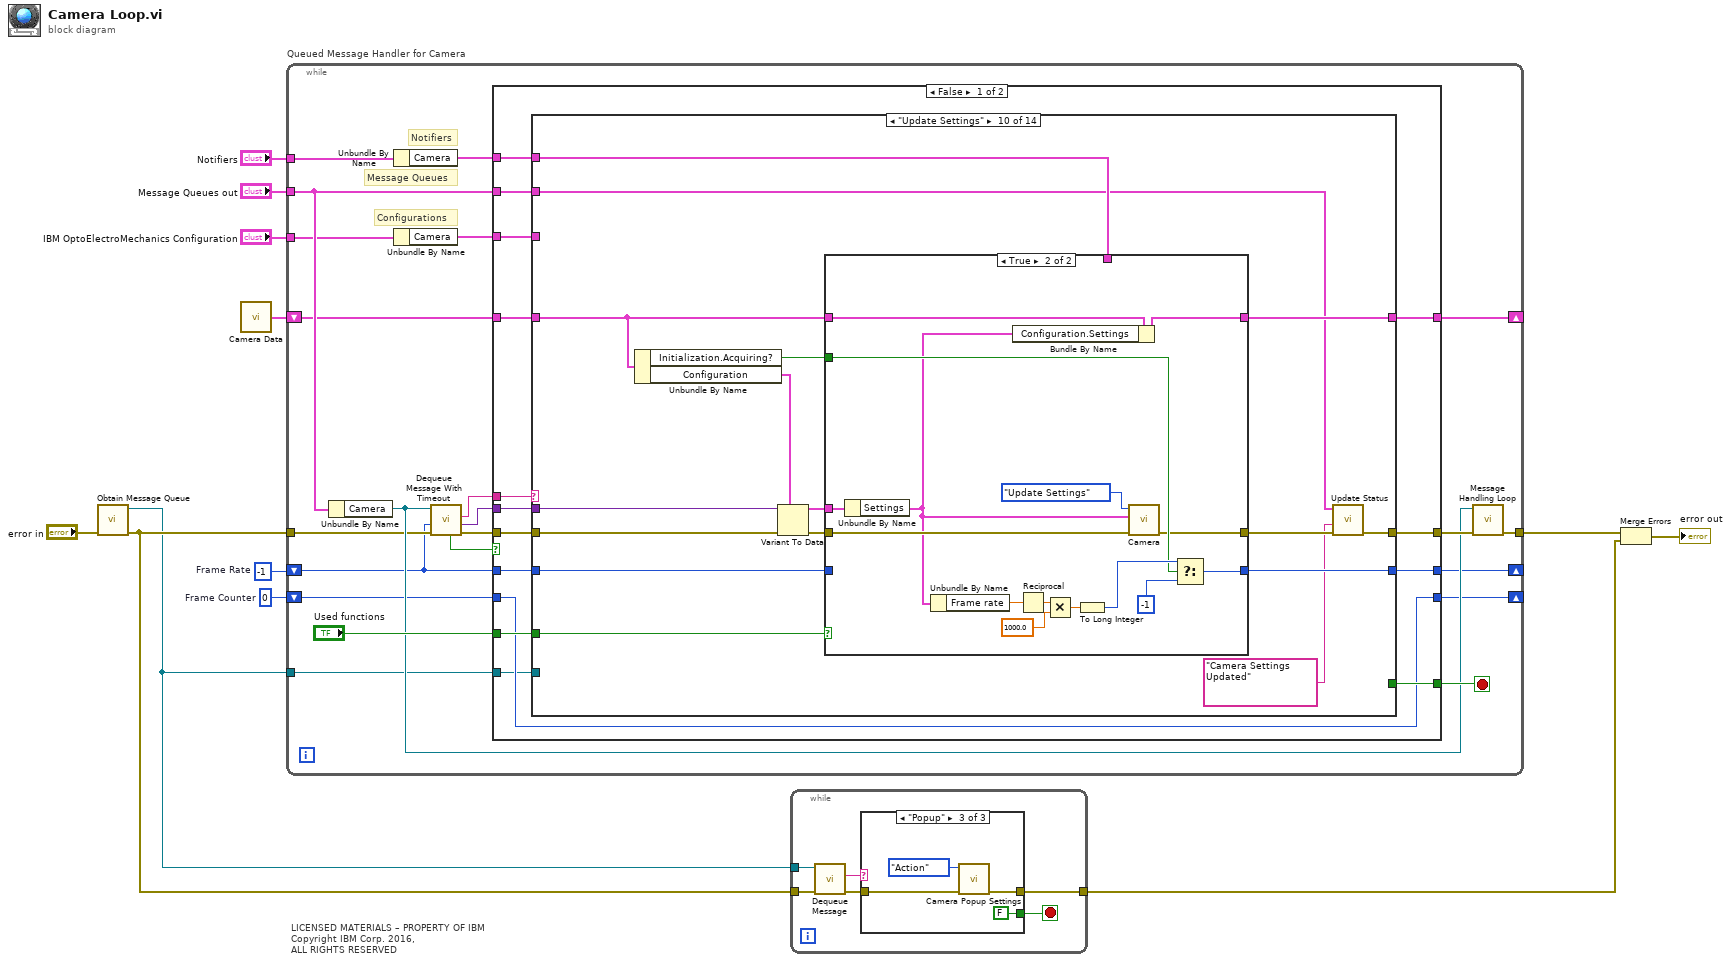
[diagram p0: block diagram]
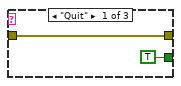
[diagram p2: hidden frame]
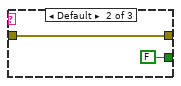
[diagram p3: hidden frame]
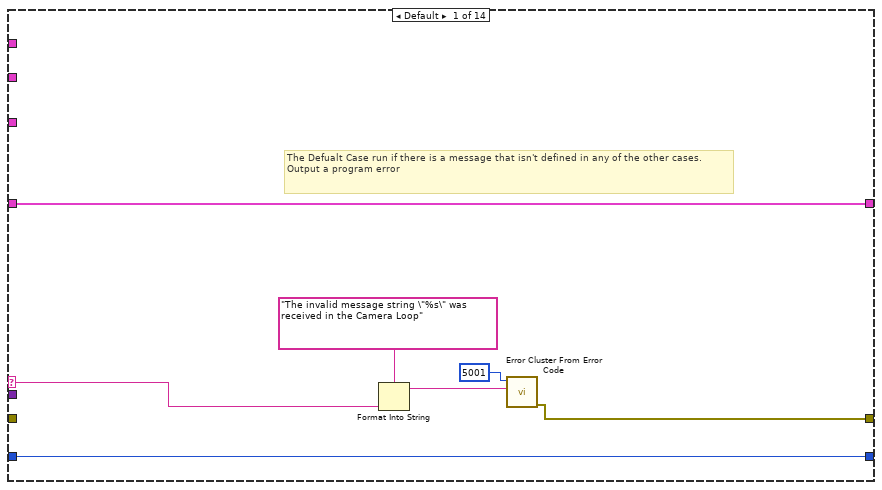
[diagram p4: hidden frame]
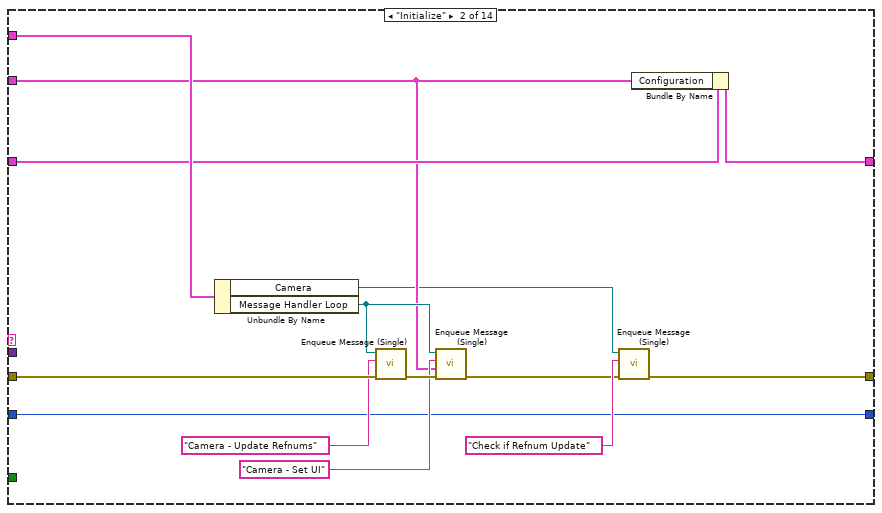
[diagram p5: hidden frame]
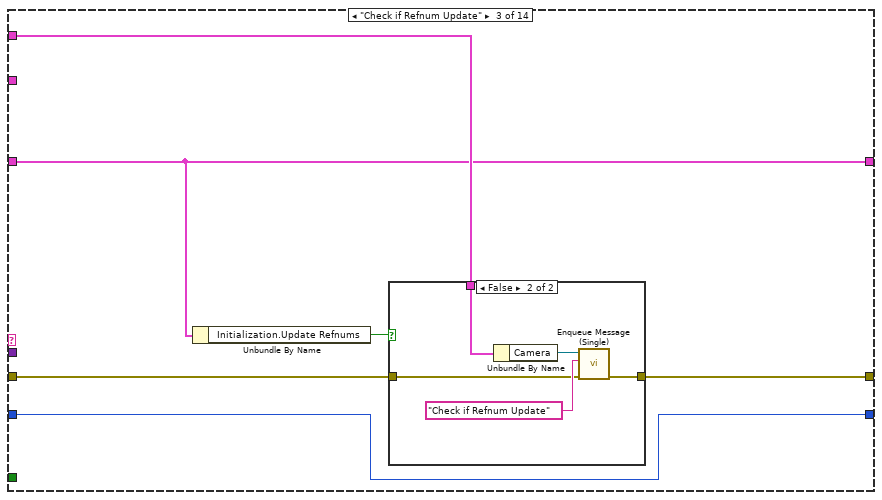
[diagram p6: hidden frame]
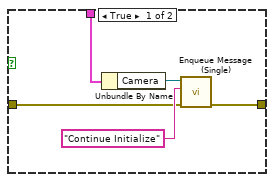
[diagram p7: hidden frame]
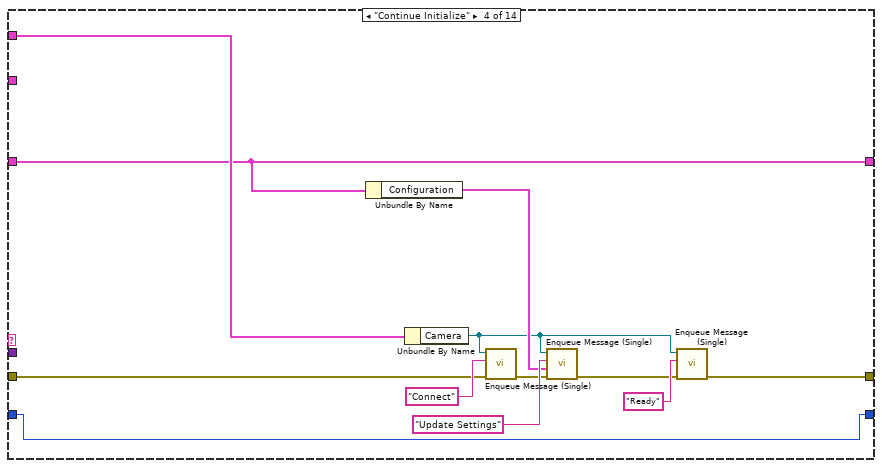
[diagram p8: hidden frame]
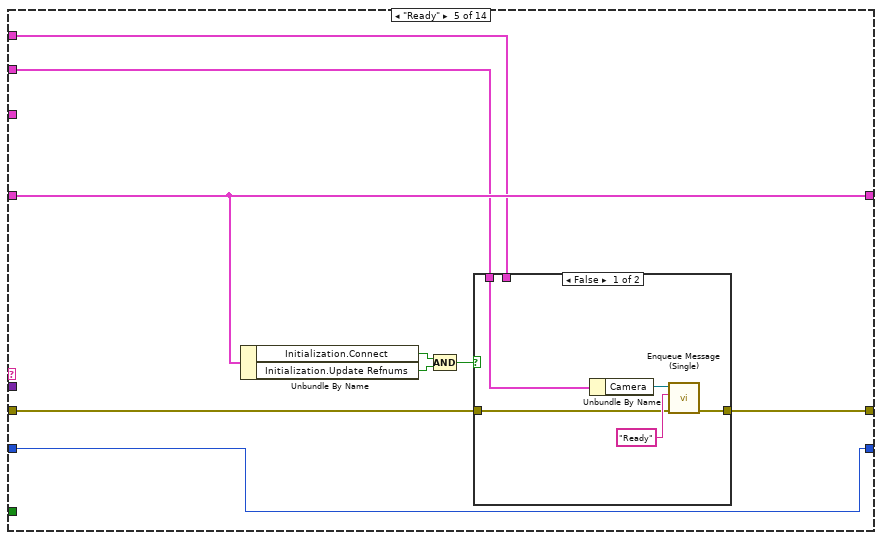
[diagram p9: hidden frame]
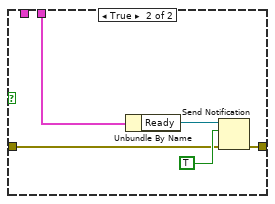
[diagram p10: hidden frame]
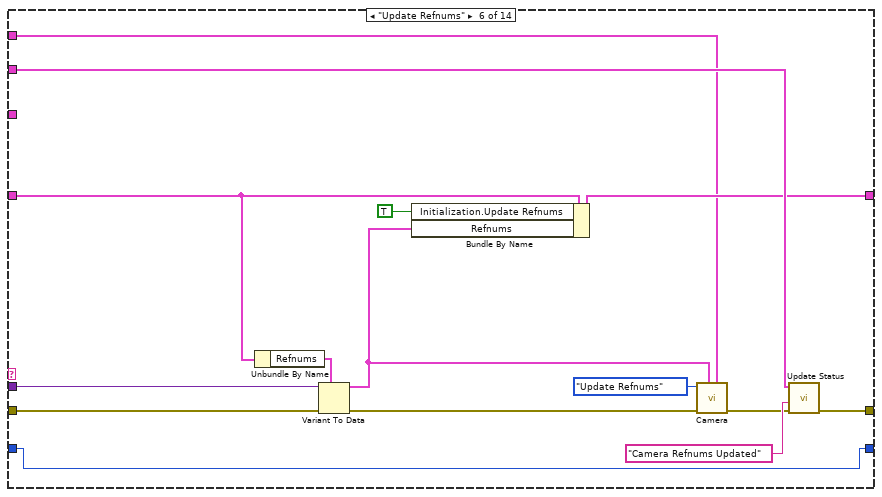
[diagram p11: hidden frame]
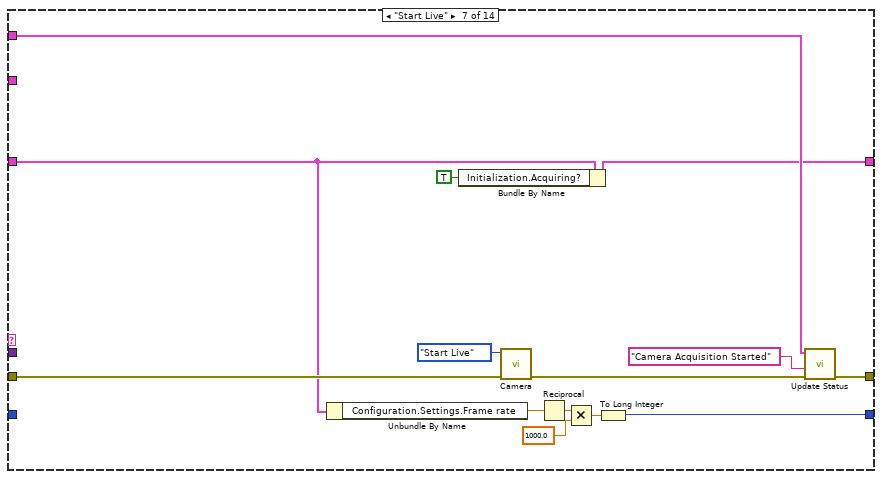
[diagram p12: hidden frame]
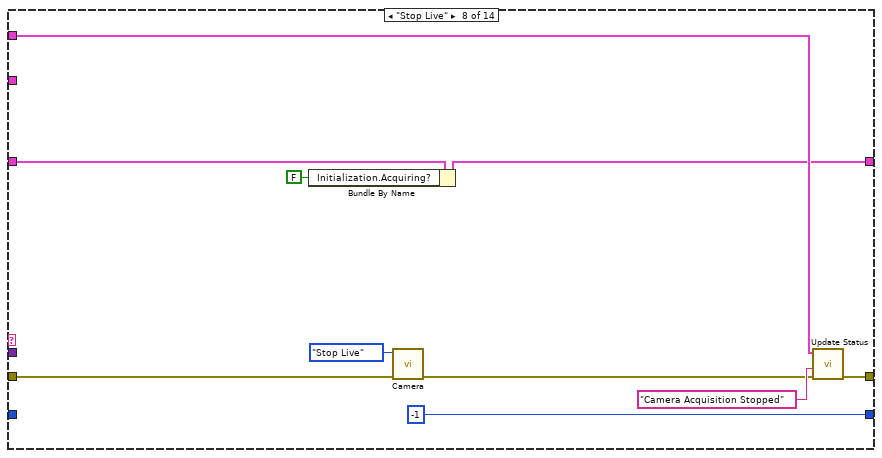
[diagram p13: hidden frame]
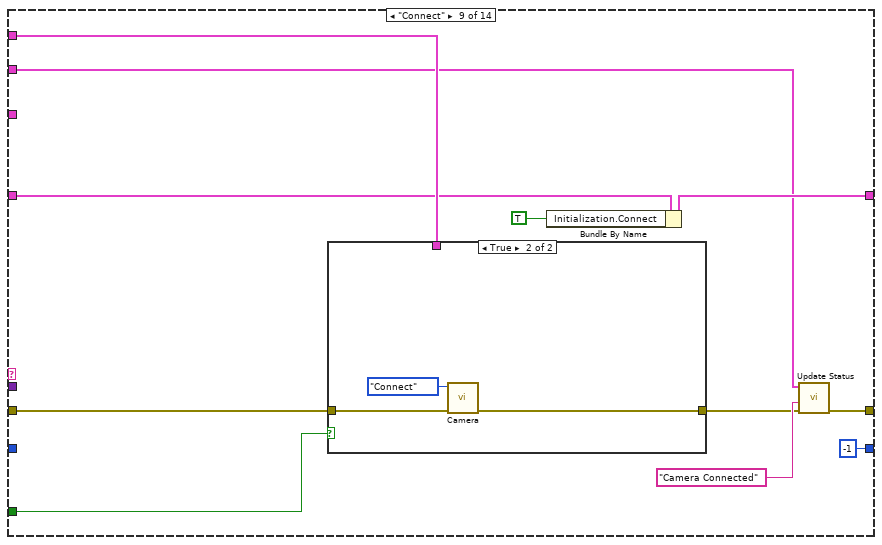
[diagram p14: hidden frame]
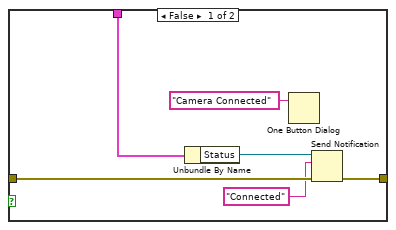
[diagram p15: hidden frame]
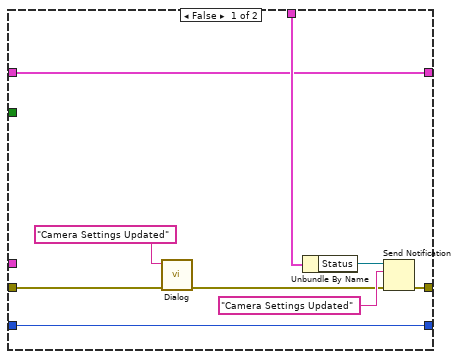
[diagram p16: hidden frame]
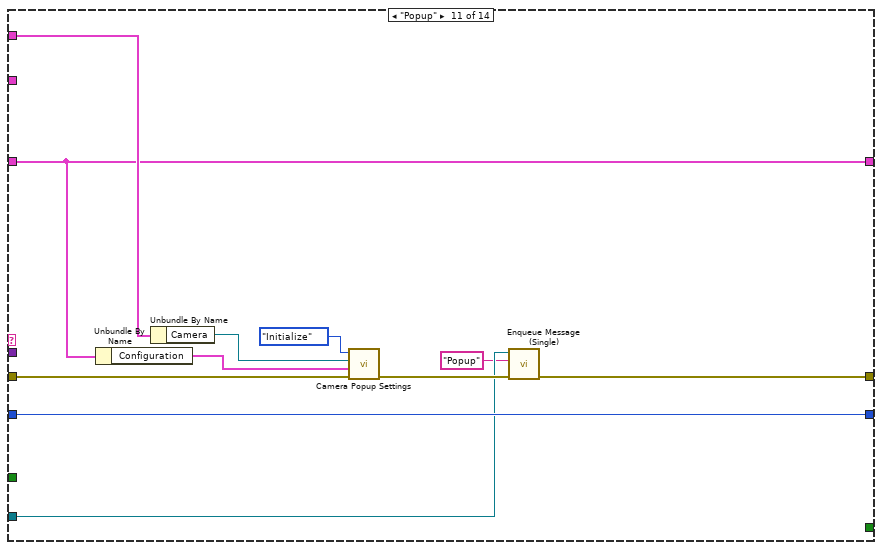
[diagram p17: hidden frame]
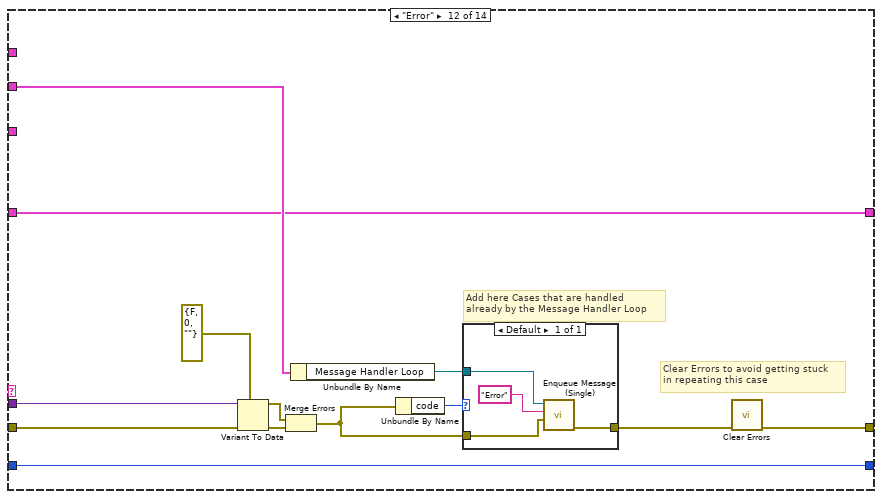
[diagram p18: hidden frame]
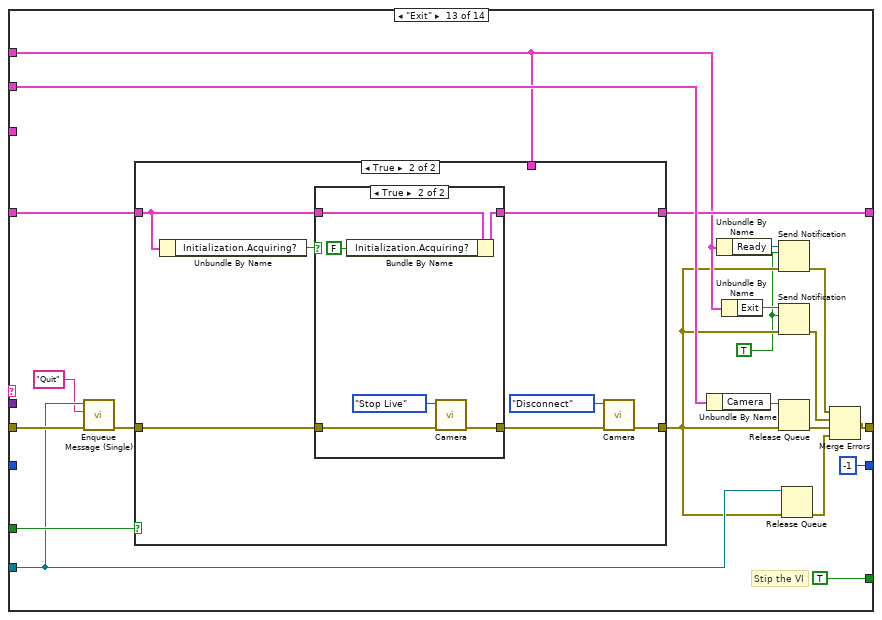
[diagram p19: hidden frame]
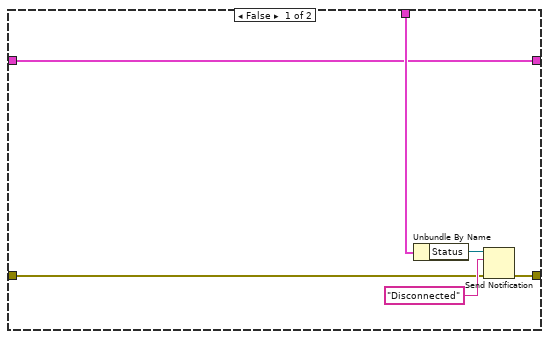
[diagram p20: hidden frame]
diagram:
  w7 = 0  # Frame Counter
  w8 = -1  # Frame Rate
  # "LICENSED MATERIALS – PROPERTY OF IBM\nCopyright IBM Corp. 2016,\nALL RIGHTS RESERVED"
  n1 = call "Obtain Message Queue.vi"("error in (no error)"="error in") -> ("error out"=w3:errorcluster, "Message Queue"=w2:refnum<queue>)  [unwired: 1 in, 8 out]
  n2 = call "Camera Data.vi"() -> ("Camera Data"=w10:T58)
  n3 = while "Queued Message Handler for Camera" {
    tunnel: w3 -> [w19]
    tunnel: [w31] -> w1
    tunnel: "Message Queues out" -> [w34]
    tunnel: "Notifiers" -> [w25]
    tunnel: "IBM OptoElectroMechanics Configuration" -> [w30]
    shift-right: [w26] -> _
    shift-left: w10 -> [w27]
    shift-right: [w16] -> _
    shift-left: w8 -> [w14]
    shift-right: [w15] -> _
    shift-left: w7 -> [w17]
    tunnel: w2 -> [w13]
    stop <- w33 stop-if-true
    # "Configurations"
    # "Notifiers"
    # "Message Queues"
    n4 = Unbundle By Name(w34) -> ("Camera"=w23:refnum<queue>)
    n5 = Unbundle By Name(w25) -> ("Camera"=w24:T51)
    n6 = Unbundle By Name(w30) -> ("Camera"=w29:T22)
    n7 = call "Dequeue Message With Timeout.vi"("error in (no error)"=w19, "Timeout in ms (-1)"=w14, "Queue In"=w23) -> ("error out"=w20:errorcluster, "Message Data"=w21:variant, "Message"=w22:string, "timed out?"=w18:bool)  [unwired: 4 in, 1 out]
    n8 = case shown="False" w18 {
      tunnel: w34 -> [w49 _]
      tunnel: [w48 _] -> w33
      tunnel: [w47 w305] -> w32
      tunnel: w29 -> [w46 _]
      tunnel: "Used functions" -> [w45 _]
      tunnel: w27 -> [w44 w294]
      tunnel: [w43 w294] -> w26
      tunnel: w24 -> [w42 _]
      tunnel: w22 -> [w41 _]
      tunnel: w21 -> [w40 _]
      tunnel: w20 -> [w39 w303]
      tunnel: w14 -> [w37 w302]
      tunnel: w17 -> [w38 w297]
      tunnel: [w36 w302] -> w16
      tunnel: [w38 w296] -> w15
      tunnel: w13 -> [w35 _]
      frame False {
        n9 = case shown="\"Update Settings\"" w41 {
          selector: w41 -> [w53 _ _ _ _ _ _ _ _ _ _ _ _ _]
          tunnel: w39 -> [_ w67 w74 w88 w103 w131 w137 w150 w162 w190 w226 w237 w252 w292]
          tunnel: [w52 w62 w75 w96 w101 w130 w146 w156 w158 w179 w219 w232 w256 w291] -> w47
          tunnel: w40 -> [_ _ _ _ _ w132 _ _ _ w192 _ w230 _ _]
          tunnel: w49 -> [_ w70 w76 w98 w102 w128 w144 w154 w160 w178 w225 w238 w261 _]
          tunnel: w42 -> [_ _ _ _ w100 w121 _ _ w166 w184 _ _ w249 w290]
          tunnel: [_ _ _ _ _ _ _ _ _ _ _ _ TRUE ("Priority Message? (F)") _] -> w48
          tunnel: w46 -> [_ w61 _ _ _ _ _ _ _ _ _ _ _ _]
          tunnel: w44 -> [w51 w69 w73 w94 w105 w125 w134 w153 w164 w186 w222 w229 w259 w287]
          tunnel: w45 -> [_ _ _ _ _ _ _ _ w167 w189 _ _ w262 _]
          tunnel: [w51 w60 w73 w94 w105 w127 w143 w152 w165 w187 w222 w229 w258 w287] -> w43
          tunnel: w37 -> [w50 w59 w71 w91 w99 w118 _ _ _ w181 w227 w228 _ w288]
          tunnel: [w50 w59 w71 w91 w99 w118 w135 -1 -1 ("Frame Rate") w182 w227 w228 -1 w288] -> w36
          tunnel: w35 -> [_ _ _ _ _ _ _ _ _ _ w218 _ w251 _]
          frame Default {
            # "The Defualt Case run if there is a message that isn't defined in any of the other cases.\nOutput a program error"
            n10 = Format Into String(format string="The invalid message string \"%s\" was  received in the Camera Loop", w53) -> (resulting string=w55:string)  [unwired: 2 in, 1 out]
            n11 = call <vilib>:"Error Cluster From Error Code.vi"("error message (\"\")"=w55, "error code (0)"=5001) -> ("error out"=w52:errorcluster)  [unwired: 2 in, 5 out]
          }
          frame "Initialize" {
            n12 = Unbundle By Name(w70) -> ("Camera"=w58:refnum<queue>, "Message Handler Loop"=w63:refnum<queue>)
            n13 = call "Enqueue Message (Single).vi"("error in (no error)"=w67, "Message"="Camera - Update Refnums", "Message Queue"=w63) -> ("error out"=w65:errorcluster)  [unwired: 1 in, 7 out]
            n14 = call "Enqueue Message (Single).vi"("error in (no error)"=w65, "Message Data"=w61, "Message"="Camera - Set UI", "Message Queue"=w63) -> ("error out"=w57:errorcluster)  [unwired: 7 out]
            n15 = call "Enqueue Message (Single).vi"("error in (no error)"=w57, "Message"="Check if Refnum Update", "Message Queue"=w58) -> ("error out"=w62:errorcluster)  [unwired: 1 in, 7 out]
            n16 = Bundle By Name(cluster=w69, "Configuration"=w61) -> (w60:T58)
          }
          frame "Check if Refnum Update" {
            n17 = Unbundle By Name(w73) -> ("Initialization.Update Refnums"=w72:bool)
            n18 = case shown="False" w72 {
              tunnel: w76 -> [w81 w86]
              tunnel: [w78 w83] -> w75
              tunnel: w74 -> [w77 w82]
              frame True {
                n19 = Unbundle By Name(w81) -> ("Camera"=w79:refnum<queue>)
                n20 = call "Enqueue Message (Single).vi"("error in (no error)"=w77, "Message"="Continue Initialize", "Message Queue"=w79) -> ("error out"=w78:errorcluster)  [unwired: 1 in, 7 out]
              }
              frame False {
                n21 = Unbundle By Name(w86) -> ("Camera"=w84:refnum<queue>)
                n22 = call "Enqueue Message (Single).vi"("error in (no error)"=w82, "Message"="Check if Refnum Update", "Message Queue"=w84) -> ("error out"=w83:errorcluster)  [unwired: 1 in, 7 out]
              }
            }
          }
          frame "Continue Initialize" {
            n23 = Unbundle By Name(w94) -> ("Configuration"=w93:T22)
            n24 = Unbundle By Name(w98) -> ("Camera"=w89:refnum<queue>)
            n25 = call "Enqueue Message (Single).vi"("error in (no error)"=w88, "Message"="Connect", "Message Queue"=w89) -> ("error out"=w87:errorcluster)  [unwired: 1 in, 7 out]
            n26 = call "Enqueue Message (Single).vi"("error in (no error)"=w87, "Message Data"=w93, "Message"="Update Settings", "Message Queue"=w89) -> ("error out"=w92:errorcluster)  [unwired: 7 out]
            n27 = call "Enqueue Message (Single).vi"("error in (no error)"=w92, "Message"="Ready", "Message Queue"=w89) -> ("error out"=w96:errorcluster)  [unwired: 1 in, 7 out]
          }
          frame "Ready" {
            n28 = Unbundle By Name(w105) -> ("Initialization.Connect"=w106:bool, "Initialization.Update Refnums"=w104:bool)
            n29 = Compound Arithmetic op=AND(w106, w104) -> (w107:bool)
            n30 = case shown="False" w107 {
              tunnel: [w110 w115] -> w101
              tunnel: w103 -> [w109 w114]
              tunnel: w102 -> [w108 _]
              tunnel: w100 -> [_ w113]
              frame False {
                n31 = Unbundle By Name(w108) -> ("Camera"=w112:refnum<queue>)
                n32 = call "Enqueue Message (Single).vi"("error in (no error)"=w109, "Message"="Ready", "Message Queue"=w112) -> ("error out"=w110:errorcluster)  [unwired: 1 in, 7 out]
              }
              frame True {
                n33 = Unbundle By Name(w113) -> ("Ready"=w116:refnum<notifier>)
                n34 = Send Notification(notification=TRUE, notifier=w116, error in (no error)=w114) -> (error out=w115:errorcluster)  [unwired: 1 out]
              }
            }
          }
          frame "Update Refnums" {
            n35 = Unbundle By Name(w125) -> ("Refnums"=w124:T59)
            n36 = Variant To Data(error in=w131, type=w124, Variant=w132) -> (data=w120:T59, error out=w123:errorcluster)
            n37 = Bundle By Name(cluster=w125, "Initialization.Update Refnums"=TRUE, "Refnums"=w120) -> (w127:T58)
            n38 = call "Camera.vi"("Camera Notifiers"=w121, "Refnums"=w120, "Error In"=w123, "Function"=Camera_Functions."Update Refnums") -> ("Error Out"=w119:errorcluster)  [unwired: 5 in, 2 out]
            n39 = call "Update Status.vi"("error in"=w119, "String"="Camera Refnums Updated" ("button name (\"OK\")"), "Message Queues out"=w128) -> ("error out"=w130:errorcluster)  [unwired: 8 out]
          }
          frame "Start Live" {
            n40 = Unbundle By Name(w134) -> ("Configuration.Settings.Frame rate"=w139:dbl)
            n41 = Bundle By Name(cluster=w134, "Initialization.Acquiring?"=TRUE ("Initialization.Acquiring")) -> (w143:T58)
            n42 = call "Camera.vi"("Error In"=w137, "Function"=Camera_Functions."Start Live") -> ("Error Out"=w136:errorcluster)  [unwired: 7 in, 2 out]
            n43 = Reciprocal(x=w139) -> (1/x=w141:dbl)
            n44 = Multiply(x=w141, y=1000.0) -> (x*y=w138:dbl)
            n45 = To Long Integer(number=w138) -> (32bit integer=w135:i32)
            n46 = call "Update Status.vi"("error in"=w136, "String"="Camera Acquisition Started" ("button name (\"OK\")"), "Message Queues out"=w144) -> ("error out"=w146:errorcluster)  [unwired: 8 out]
          }
          frame "Stop Live" {
            n47 = Bundle By Name(cluster=w153, "Initialization.Acquiring?"=FALSE ("Initialization.Acquiring")) -> (w152:T58)
            n48 = call "Camera.vi"("Error In"=w150, "Function"=Camera_Functions."Stop Live") -> ("Error Out"=w149:errorcluster)  [unwired: 7 in, 2 out]
            n49 = call "Update Status.vi"("error in"=w149, "String"="Camera Acquisition Stopped" ("button name (\"OK\")"), "Message Queues out"=w154) -> ("error out"=w156:errorcluster)  [unwired: 8 out]
          }
          frame "Connect" {
            n50 = case shown="True" w167 {
              tunnel: w162 -> [w171 w175]
              tunnel: [w170 w174] -> w159
              tunnel: w166 -> [w173 _]
              frame False {
                n51 = Unbundle By Name(w173) -> ("Status"=w172:refnum<notifier>)
                n52 = One Button Dialog(message="Camera Connected" ("button name (\"OK\")")) -> ()  [unwired: 2 out]
                n53 = Send Notification(notification="Connected", notifier=w172, error in (no error)=w171) -> (error out=w170:errorcluster)  [unwired: 1 out]
              }
              frame True {
                n54 = call "Camera.vi"("Error In"=w175, "Function"=Camera_Functions."Connect") -> ("Error Out"=w174:errorcluster)  [unwired: 7 in, 2 out]
              }
            }
            n55 = Bundle By Name(cluster=w164, "Initialization.Connect"=TRUE ("Initialization.Update Visa Session")) -> (w165:T58)
            n56 = call "Update Status.vi"("error in"=w159, "String"="Camera Connected" ("button name (\"OK\")"), "Message Queues out"=w160) -> ("error out"=w158:errorcluster)  [unwired: 8 out]
          }
          frame "Update Settings" {
            n57 = Unbundle By Name(w186) -> ("Initialization.Acquiring?"=w183:bool, "Configuration"=w185:T22)
            n58 = Variant To Data(error in=w190, type=w185, Variant=w192) -> (data=w188:T22, error out=w191:errorcluster)
            n59 = case shown="True" w189 {
              tunnel: w191 -> [w198 w204]
              tunnel: [w196 w205] -> w180
              tunnel: w188 -> [_ w203]
              tunnel: w186 -> [w194 w216]
              tunnel: [w194 w215] -> w187
              tunnel: w184 -> [w195 _]
              tunnel: w183 -> [_ w208]
              tunnel: [w193 w207] -> w182
              tunnel: w181 -> [w193 _]
              frame False {
                n60 = call "Dialog.vi"("error in (no error)"=w198, "message"="Camera Settings Updated" ("button name (\"OK\")")) -> ("error out"=w197:errorcluster)  [unwired: 1 in, 8 out]
                n61 = Unbundle By Name(w195) -> ("Status"=w199:refnum<notifier>)
                n62 = Send Notification(notification="Camera Settings Updated", notifier=w199, error in (no error)=w197) -> (error out=w196:errorcluster)  [unwired: 1 out]
              }
              frame True {
                n63 = Unbundle By Name(w203) -> ("Settings"=w202:T23)
                n64 = Unbundle By Name(w202) -> ("Frame rate"=w210:dbl)
                n65 = Bundle By Name(cluster=w216, "Configuration.Settings"=w202) -> (w215:T58)
                n66 = Reciprocal(x=w210) -> (1/x=w214:dbl)
                n67 = Multiply(x=w214, y=1000.0) -> (x*y=w211:dbl)
                n68 = To Long Integer(number=w211) -> (32bit integer=w212:i32)
                n69 = call "Camera.vi"("Error In"=w204, "Settings"=w202, "Function"=Camera_Functions."Update Settings") -> ("Error Out"=w205:errorcluster)  [unwired: 6 in, 2 out]
                n70 = Select(t=w212, s=w208, f=-1) -> (s? t:f=w207:i32)
              }
            }
            n71 = call "Update Status.vi"("error in"=w180, "String"="Camera Settings Updated" ("button name (\"OK\")"), "Message Queues out"=w178) -> ("error out"=w179:errorcluster)  [unwired: 8 out]
          }
          frame "Popup" {
            n72 = Unbundle By Name(w222) -> ("Configuration"=w221:T22)
            n73 = Unbundle By Name(w225) -> ("Camera"=w224:refnum<queue>)
            n74 = call "Camera Popup Settings.vi"("error in (no error)"=w226, "Camera Configuration"=w221, "Camera"=w224, "Function"=enum16{"Initialize", "Action"}."Initialize") -> ("error out"=w223:errorcluster)  [unwired: 7 in]
            n75 = call "Enqueue Message (Single).vi"("error in (no error)"=w223, "Message"="Popup", "Message Queue"=w218) -> ("error out"=w219:errorcluster)  [unwired: 7 in, 1 out]
          }
          frame "Error" {
            # "Clear Errors to avoid getting stuck \nin repeating this case"
            # "Add here Cases that are handled \nalready by the Message Handler Loop"
            n76 = Variant To Data(error in=w237, type=errorcluster {"status"=FALSE, "code"=0, "source"=""} ("error out"), Variant=w230) -> (data=w236:errorcluster, error out=w235:errorcluster)
            n77 = Merge Errors(w236, w235) -> (w234:errorcluster)
            n78 = Unbundle By Name(w238) -> ("Message Handler Loop"=w240:refnum<queue>)
            n79 = Unbundle By Name(w234) -> ("code"=w231:i32)
            n80 = case shown="Default" w231 {
              tunnel: w240 -> [w244]
              tunnel: w234 -> [w242]
              tunnel: [w241] -> w233
              frame Default {
                n81 = call "Enqueue Message (Single).vi"("Message Data"=w242, "Message"="Error", "Message Queue"=w244) -> ("error out"=w241:errorcluster)  [unwired: 1 in, 7 out]
              }
            }
            n82 = call <vilib>:"Clear Errors.vi"("error in (no error)"=w233) -> ("error out"=w232:errorcluster)  [unwired: 1 in, 5 out]
          }
          frame "Exit" {
            w245 = TRUE ("Priority Message? (F)")
            # "Stip the VI"
            n83 = call "Enqueue Message (Single).vi"("error in (no error)"=w252, "Message"="Quit", "Message Queue"=w251) -> ("error out"=w253:errorcluster)  [unwired: 7 in, 1 out]
            n84 = case shown="True" w262 {
              tunnel: w253 -> [w269 w272]
              tunnel: [w268 w276] -> w247
              tunnel: w249 -> [w267 _]
              tunnel: w259 -> [w266 w274]
              tunnel: [w266 w275] -> w258
              frame False {
                n85 = Unbundle By Name(w267) -> ("Status"=w270:refnum<notifier>)
                n86 = Send Notification(notification="Disconnected", notifier=w270, error in (no error)=w269) -> (error out=w268:errorcluster)  [unwired: 1 out]
              }
              frame True {
                n87 = Unbundle By Name(w274) -> ("Initialization.Acquiring?"=w273:bool)
                n88 = case shown="True" w273 {
                  tunnel: [w280 w286] -> w277
                  tunnel: w272 -> [w280 w285]
                  tunnel: w274 -> [w279 w284]
                  tunnel: [w279 w283] -> w275
                  frame False {
                  }
                  frame True {
                    n89 = Bundle By Name(cluster=w284, "Initialization.Acquiring?"=FALSE) -> (w283:T58)
                    n90 = call "Camera.vi"("Error In"=w285, "Function"=Camera_Functions."Stop Live") -> ("Error Out"=w286:errorcluster)  [unwired: 7 in, 2 out]
                  }
                }
                n91 = call "Camera.vi"("Error In"=w277, "Function"=Camera_Functions."Disconnect") -> ("Error Out"=w276:errorcluster)  [unwired: 7 in, 2 out]
              }
            }
            n92 = Unbundle By Name(w261) -> ("Camera"=w265:refnum<queue>)
            n93 = Unbundle By Name(w249) -> ("Ready"=w248:refnum<notifier>)
            n94 = Unbundle By Name(w249) -> ("Exit"=w264:refnum<notifier>)
            n95 = Send Notification(notification=w245, notifier=w248, error in (no error)=w247) -> (error out=w246:errorcluster)  [unwired: 1 out]
            n96 = Send Notification(notification=w245, notifier=w264, error in (no error)=w247) -> (error out=w255:errorcluster)  [unwired: 1 out]
            n97 = Release Queue(queue=w265, error in (no error)=w247) -> (error out=w257:errorcluster)  [unwired: 3 out]
            n98 = Release Queue(queue=w251, error in (no error)=w247) -> (error out=w254:errorcluster)  [unwired: 1 in, 2 out]
            n99 = Merge Errors(w246, w255, w257, w254) -> (w256:errorcluster)
          }
          frame "Notify Status" {
            n100 = Unbundle By Name(w290) -> ("Instrument Data"=w289:refnum<notifier>)
            n101 = Send Notification(notification=w287, notifier=w289, error in (no error)=w292) -> (error out=w291:errorcluster)  [unwired: 1 out]
          }
        }
      }
      frame True {
        n102 = Quotient & Remainder(x=w297, y=10) -> (x-y*floor(x/y)=w299:i32)  [unwired: 1 out]
        n103 = Equal To 0?(x=w299) -> (x = 0?=w295:bool)
        n104 = Unbundle By Name(w294) -> ("Configuration.Settings"=w293:T23)
        n105 = Increment(x=w297) -> (x+1=w300:i32)
        n106 = Select(t=0, s=w295, f=w300) -> (s? t:f=w296:i32)
        n107 = case shown="True" w295 {
          tunnel: w303 -> [w307 w311]
          tunnel: [w307 w310] -> w304
          tunnel: w293 -> [_ w308]
          frame False {
          }
          frame True {
            n108 = call "Camera.vi"("Error In"=w311, "Settings"=w308, "Function"=Camera_Functions."Update Settings") -> ("Error Out"=w310:errorcluster)  [unwired: 6 in, 2 out]
          }
        }
        n109 = call "Camera.vi"("Error In"=w304, "Function"=Camera_Functions."Acquire") -> ("Error Out"=w305:errorcluster)  [unwired: 7 in, 2 out]
      }
    }
    n110 = call "Message Handling Loop.vi"("error in (no error)"=w32, "Message Queue"=w23) -> ("dup error in"=w31:errorcluster)  [unwired: 9 out]
  }
  n111 = while {
    tunnel: w2 -> [w316]
    tunnel: [w315] -> w6
    tunnel: w3 -> [w313]
    stop <- w312 stop-if-true
    n112 = call "Dequeue Message.vi"("error in (no error)"=w313, "Message Queue"=w316) -> ("error out"=w317:errorcluster, "Message"=w314:string)  [unwired: 6 in, 2 out]
    n113 = case shown="\"Popup\"" w314 {
      tunnel: w317 -> [w319 w320 w325]
      tunnel: [w319 w320 w324] -> w315
      tunnel: [TRUE FALSE FALSE] -> w312
      frame "Quit" {
      }
      frame Default {
      }
      frame "Popup" {
        n114 = call "Camera Popup Settings.vi"("error in (no error)"=w325, "Function"=enum16{"Initialize", "Action"}."Action") -> ("error out"=w324:errorcluster)  [unwired: 9 in]
      }
    }
  }
  n115 = Merge Errors(w1, w6) -> (→"error out":errorcluster)
